vi "QTrkQueueFramePtr.vi"(0 "QTrk Instance":T2, 1 "frame#":u32, 2 "Read timestamp from first 4 pixels (F)":bool, 3 "timestamp":u32, 4 "width":i32, 5 "height":i32, 6 "Pixel data type":T1=enum."QTrkU16", 7 "ROI Positions (corner-based)":cluster{"X":i32, "Y":i32}[](array[cluster]), 8 "Image pitch\n(bytes per row)":i32, 9 "ZLUT Index offset (0)":i32, 11 "Image Pointer":u64) -> (14 "QTrk Instance (out)":T2, 19 "error out":errorcluster)   [LabVIEW 2011]
uses:
  QTrkInstance.ctl
  QTrkPixelDataType.ctl
  QTrkLocalizationJob.ctl
  XYZf.ctl
  QTrkDLL.vi
panel:
  out "timestamp from frame":u32
  in  "zlutPlane (0)":i32
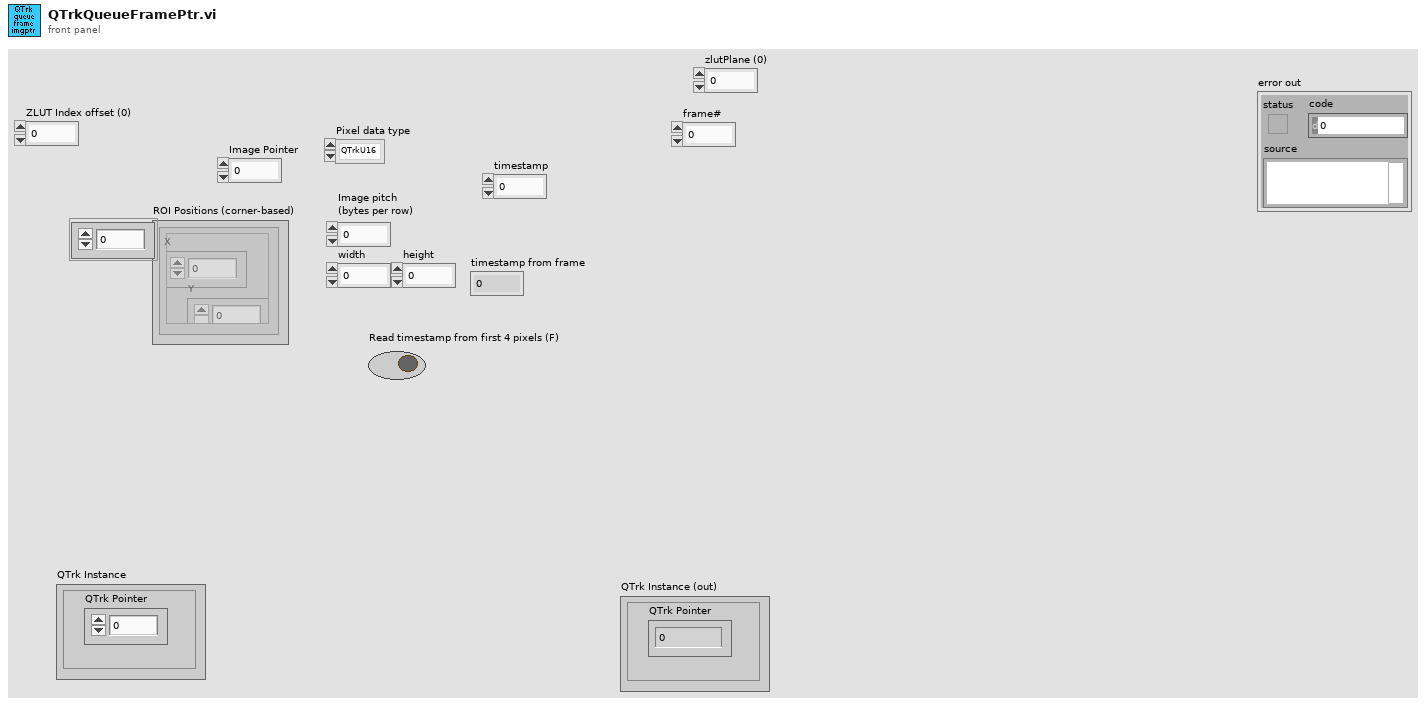
[diagram p1: front panel]
types:
  T1 = typedef "QTrkPixelDataType.ctl" = enum16{"QTrkU8", "QTrkU16", "QTrkFloat"}
  T2 = typedef "QTrkInstance.ctl" = cluster{"QTrk Pointer":u64}
  T3 = typedef "QTrkLocalizationJob.ctl" = cluster{"Frame#":u32, "Timestamp":u32, "ZLUT Index / bead#":i32, "ZLUT Plane":i32, "Initial guess":T4}
  T4 = typedef "XYZf.ctl" = cluster{"X":sgl, "Y":sgl, "Z":sgl}
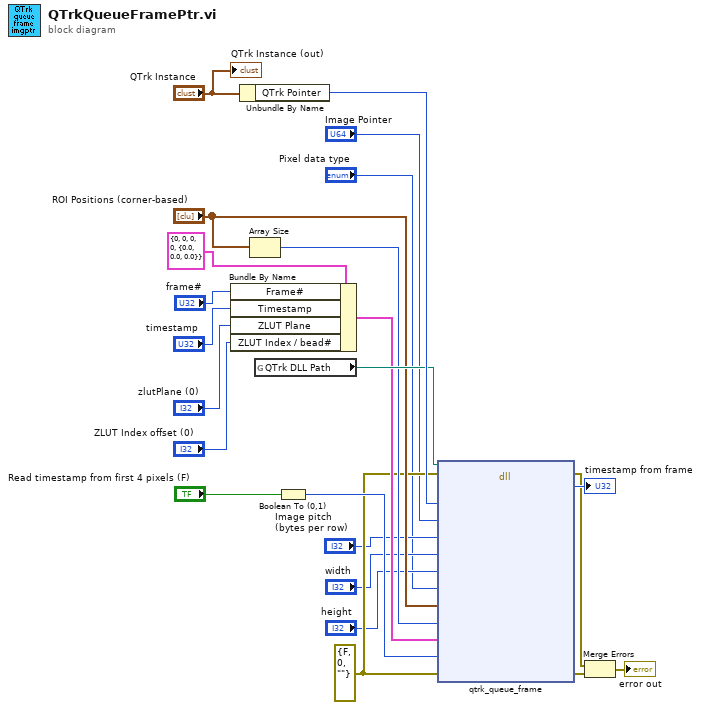
[diagram p0: block diagram]
diagram:
  w7 = errorcluster {"status"=FALSE, "code"=0, "source"=""} ("error in (no error)")
  n1 = Bundle By Name(cluster=T3 {"Frame#"=0, "Timestamp"=0, "ZLUT Index / bead#"=0, "ZLUT Plane"=0, "Initial guess"={"X"=0.0, "Y"=0.0, "Z"=0.0}} ("Queue Params"), "Frame#"="frame#", "Timestamp"="timestamp", "ZLUT Plane"="zlutPlane (0)", "ZLUT Index / bead#"="ZLUT Index offset (0)") -> (w14:T3)
  n2 = Unbundle By Name("QTrk Instance") -> ("QTrk Pointer"=w22:u64)
  n3 = Array Size(array="ROI Positions (corner-based)") -> (size(s)=w20:i32)
  n4 = global read "QTrkDLL.vi" "QTrk DLL Path"() -> (w21:path)
  n5 = Boolean To (0,1)(Boolean="Read timestamp from first 4 pixels (F)") -> (0, 1=w8:i16)
  n6 = dll-call lib="D:/jcnossen1/cudaqi-tracker/bin/jtrk-labview.dll" fn="qtrk_queue_frame"(path in=w21, error in=w7, "tracker"=w22, "image"="Image Pointer", "pitch"="Image pitch\n(bytes per row)", "width"="width", "height"="height", "pixelFormat"="Pixel data type", "positions"="ROI Positions (corner-based)", "numROI"=w20, "jobInfo"=w14, "flags"=w8, "err"=w7) -> (error out=w11:errorcluster, "timestamp from frame"=→"timestamp from frame":u32, "err"=w10:errorcluster)  [unwired: 11 in, 1 out]
  n7 = Merge Errors(w11, w10) -> (→"error out":errorcluster)
  "QTrk Instance (out)" <- "QTrk Instance"
